vi "RPi_pico_Bot.vi"() -> ()   [LabVIEW 2023]
panel:
  in  "Stop (F)":bool
  out "Image Out":T1(plugin-control)
  in  "Right":bool
  in  "Left":bool
  in  "Backward":bool
  in  "Forward":bool
  in  "stop":bool
  in  "VISA resource name":refnum<visa-resource-name>
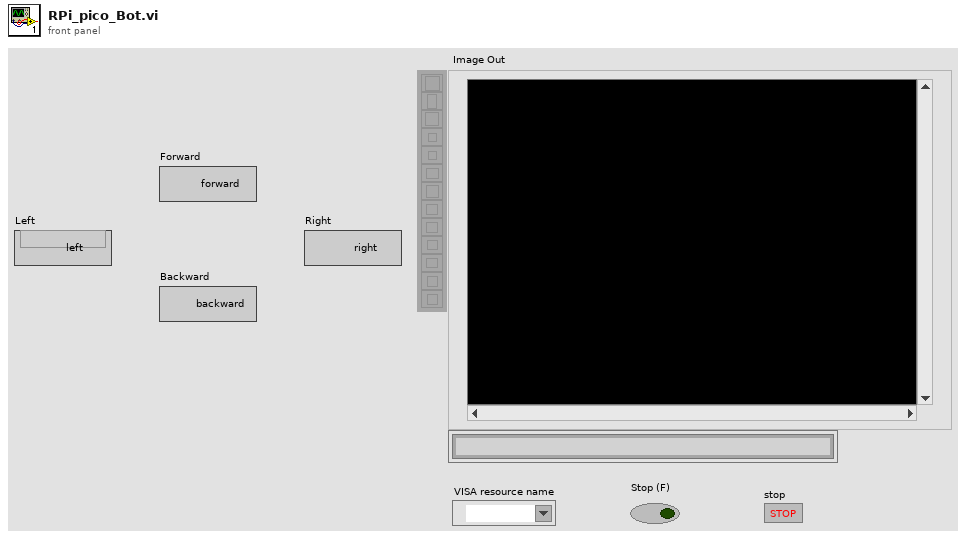
[diagram p1: front panel]
types:
  T1 = typedef "IMAQ Image.ctl" = refnum<image>
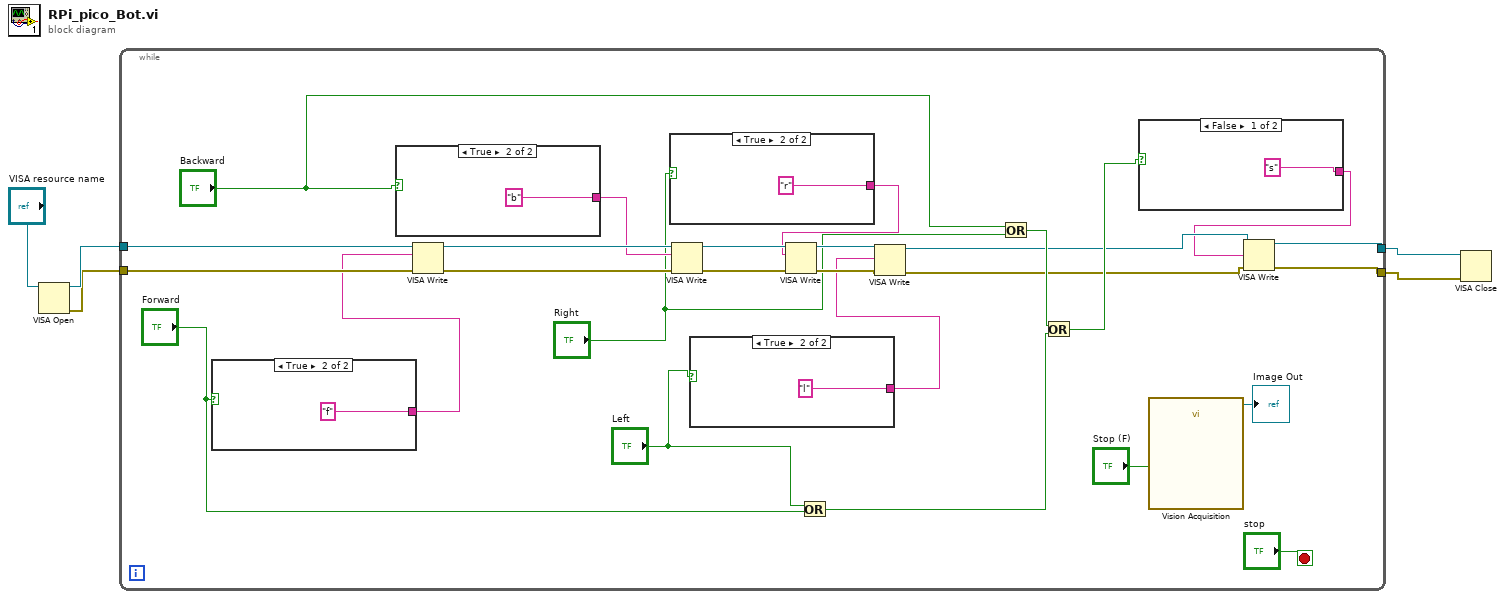
[diagram p0: block diagram]
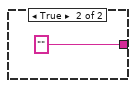
[diagram p2: hidden frame]
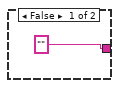
[diagram p3: hidden frame]
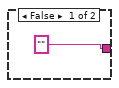
[diagram p4: hidden frame]
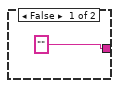
[diagram p5: hidden frame]
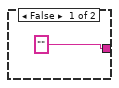
[diagram p6: hidden frame]
diagram:
  n1 = VISA Open(VISA resource name="VISA resource name") -> (VISA resource name=w5:refnum<visa-resource-name>, error out=w4:errorcluster)  [unwired: 4 in]
  n2 = while {
    tunnel: w5 -> [w32]
    tunnel: w4 -> [w31]
    tunnel: [w10] -> w2
    tunnel: [w9] -> w1
    stop <- "stop" stop-if-true
    n3 = case shown="True" "Forward" {
      tunnel: ["" "f"] -> w26
      frame False {
      }
      frame True {
      }
    }
    n4 = case shown="True" "Backward" {
      tunnel: ["" "b"] -> w27
      frame False {
      }
      frame True {
      }
    }
    n5 = VISA Write(VISA resource name=w32, write buffer=w26, error in (no error)=w31) -> (VISA resource name out=w29:refnum<visa-resource-name>, error out=w28:errorcluster)  [unwired: 1 out]
    n6 = case shown="True" "Right" {
      tunnel: ["" "r"] -> w21
      frame False {
      }
      frame True {
      }
    }
    n7 = VISA Write(VISA resource name=w29, write buffer=w27, error in (no error)=w28) -> (VISA resource name out=w25:refnum<visa-resource-name>, error out=w24:errorcluster)  [unwired: 1 out]
    n8 = case shown="True" "Left" {
      tunnel: ["" "l"] -> w20
      frame False {
      }
      frame True {
      }
    }
    n9 = VISA Write(VISA resource name=w25, write buffer=w21, error in (no error)=w24) -> (VISA resource name out=w23:refnum<visa-resource-name>, error out=w22:errorcluster)  [unwired: 1 out]
    n10 = Or(x="Left", y="Forward") -> (x .or. y?=w15:bool)
    n11 = VISA Write(VISA resource name=w23, write buffer=w20, error in (no error)=w22) -> (VISA resource name out=w12:refnum<visa-resource-name>, error out=w11:errorcluster)  [unwired: 1 out]
    n12 = Or(x="Backward", y="Right") -> (x .or. y?=w14:bool)
    n13 = Or(x=w14, y=w15) -> (x .or. y?=w13:bool)
    n14 = case shown="False" w13 {
      tunnel: ["s" ""] -> w8
      frame False {
      }
      frame True {
      }
    }
    n15 = call "Vision Acquisition"("Stop (F)"="Stop (F)") -> ("Image Out"=→"Image Out":T1)  [unwired: 24 in, 2 out]
    n16 = VISA Write(VISA resource name=w12, write buffer=w8, error in (no error)=w11) -> (VISA resource name out=w10:refnum<visa-resource-name>, error out=w9:errorcluster)  [unwired: 1 out]
  }
  n17 = VISA Close(VISA resource name=w2, error in (no error)=w1) -> ()  [unwired: 1 out]
